vi "Constants.vi"() -> ()   [LabVIEW 2017, in "Data Sharing Framework Shared.lvlib"]
doc: "Use this Global VI to access the GUIDs assigned to the page resources of the Custom Device."
uses:
  Data Sharing Framework Shared.lvlib
panel:
  in  "Tab Control":enum32{"GUIDS", "Constants", "Properties"}(tab)
  in  "Data Sharing Framework":string="37c56d03-17da-482b-8988-568955beadf2"
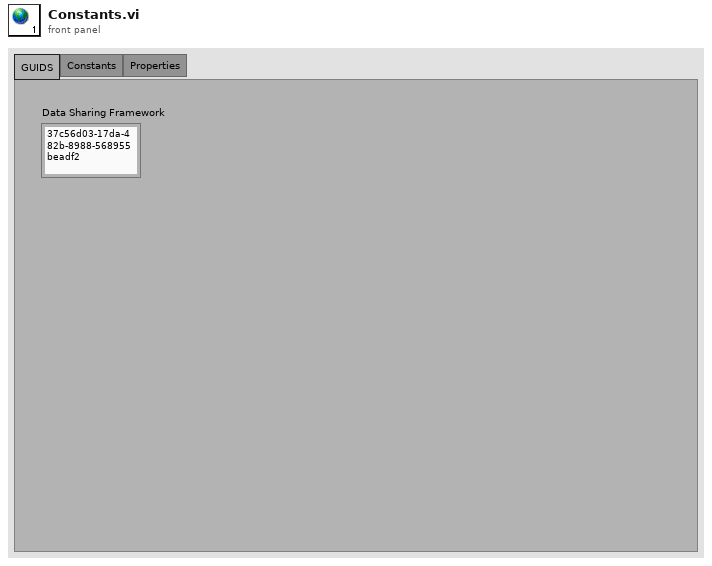
[diagram p1: front panel]
diagram:
